vi "Better Joystick.vi"(2 "Steering":i32, 3 "Lidar":i32, 5 "Drive":i32) -> (0 "Numeric 6":fxp<+/-,19,4> format="%.17g", 1 "Numeric 5":fxp<+/-,19,4> format="%.17g", 4 "Numeric 7":fxp<+/-,19,4> format="%.17g", 6 "setpoint":i32, 7 "Numeric":i32, 8 "Numeric 3":i32, 9 "Trig":bool)   [LabVIEW 2010]
uses:
  4-High Neurons/4.1.0-Datatype Typedef.ctl
  3.0-Global.vi
panel:
  in  "Lidar G":i32
  in  "Steer G":i32
  in  "Drive G":i32
  out "Pitch":i32
  out "Roll":i32
  out "Left":i32
  out "Lidar Command":i32
  out "Steering Command":i32
  out "Drive Command":i32
  in  "Magic Number for Lidar Zero Point":i32
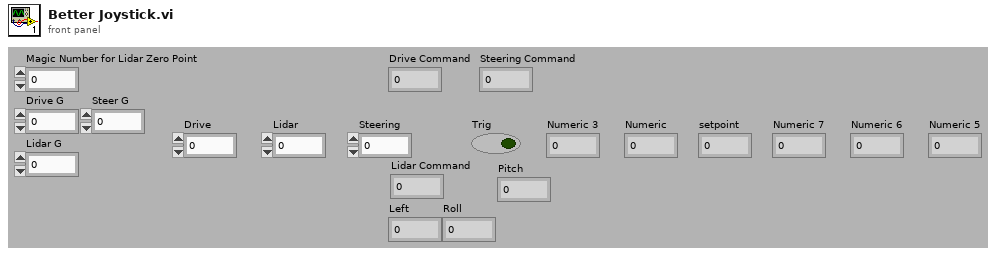
[diagram p1: front panel]
types:
  T1 = typedef "4.1.0-Datatype Typedef.ctl" = enum16{"4.1.0-Empty Data", "4.1.1-Joystick Data", "4.1.2-Behavioral Data"}
  T2 = typedef "4.1-Act Control Typedef.ctl" = cluster{"4.1.0 Data":variant, "Type of Data":T1, "E-Stop":bool, "Restart":bool, "New IP":bool, "Begin":bool, "Time":i32, "Shutdown":bool}
  T3 = typedef "4.1.1-Act Joystick.ctl" = cluster{"Trig":bool, "2":bool, "3":bool, "4":bool, "5":bool, "6":bool, "7":bool, "8":bool, "9":bool, "10":bool, "11":bool, "Pitch":i32, "Ang":bool[], "Wheel":dbl, "Roll":i32, "Yaw":i32, "Left":i32, "Right":i32}
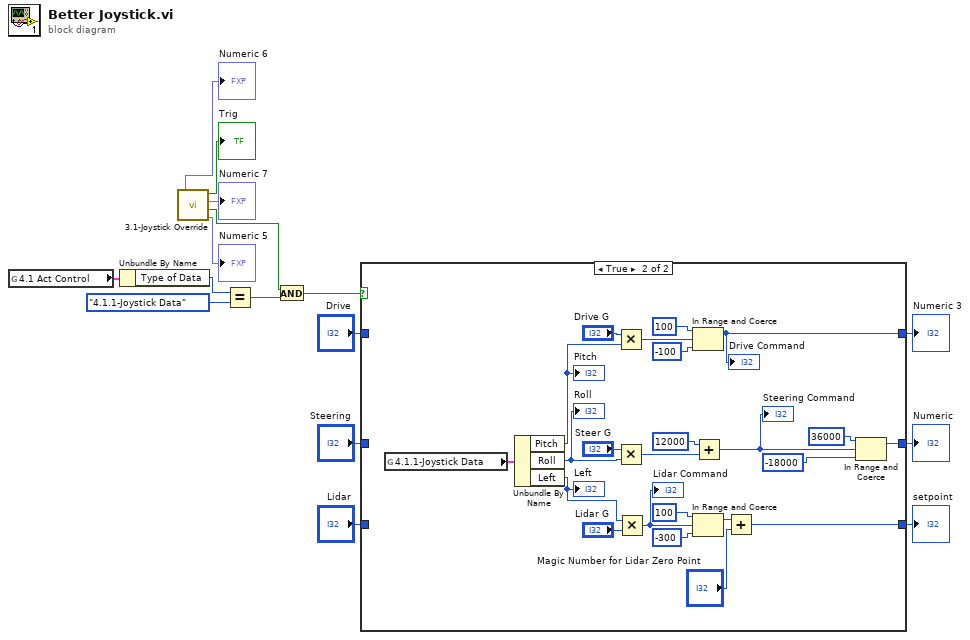
[diagram p0: block diagram]
diagram:
  n1 = global read "3.0-Global.vi" "4.1 Act Control"() -> (w5:T2)
  n2 = Unbundle By Name(w5) -> ("Type of Data"=w4:T1)
  n3 = call "3.1-Joystick Override.vi"() -> ("Numeric 2"=→"Numeric 6":fxp<+/-,19,4>, "Numeric"=→"Numeric 5":fxp<+/-,19,4>, "Joystick Setpoints"=w6:bool, "Numeric 3"=→"Numeric 7":fxp<+/-,19,4>, "Trig"=→"Trig":bool)
  n4 = Equal?(x=w4, y=4.1.0-Datatype_Typedef."4.1.1-Joystick Data") -> (x = y?=w1:bool)
  n5 = And(x=w6, y=w1) -> (x .and. y?=w2:bool)
  n6 = case shown="True" w2 {
    tunnel: [w19 w20] -> w12
    tunnel: "Drive" -> [w19 _]
    tunnel: [w18 w39] -> w14
    tunnel: "Steering" -> [w18 _]
    tunnel: [w17 w33] -> w16
    tunnel: "Lidar" -> [w17 _]
    frame False {
    }
    frame True {
      n7 = global read "3.0-Global.vi" "4.1.1-Joystick Data"() -> (w42:T3)
      n8 = Unbundle By Name(w42) -> ("Pitch"=w31:i32, "Roll"=w27:i32, "Left"=w25:i32)
      "Left" <- w25
      "Roll" <- w27
      "Pitch" <- w31
      n9 = Multiply(x="Drive G", y=w31) -> (x*y=w30:i32)
      n10 = Multiply(x="Steer G", y=w27) -> (x*y=w28:i32)
      n11 = Multiply(x=w25, y="Lidar G") -> (x*y=w24:i32)
      "Lidar Command" <- w24
      n12 = In Range and Coerce(upper limit=100, x=w30, lower limit=-100) -> (coerced(x)=w20:i32)  [unwired: 1 out]
      "Drive Command" <- w20
      n13 = In Range and Coerce(upper limit=100, x=w24, lower limit=-300) -> (coerced(x)=w34:i32)  [unwired: 1 out]
      n14 = Add(x=12000, y=w28) -> (x+y=w21:i32)
      "Steering Command" <- w21
      n15 = Add(x=w34, y="Magic Number for Lidar Zero Point") -> (x+y=w33:i32)
      n16 = In Range and Coerce(upper limit=36000, x=w21, lower limit=-18000) -> (coerced(x)=w39:i32)  [unwired: 1 out]
    }
  }
  "setpoint" <- w16
  "Numeric" <- w14
  "Numeric 3" <- w12
